vi "Generate_REF_Waveforms.vi"(8 "error in (no error)":errorcluster, 9 "sampling info":cluster{"Fs":dbl, "#s":dbl}={"Fs"=1000.0, "#s"=1000.0} {"Fs" format="%.2p"}, 10 "reset signal":bool, 11 "lockin config":T1 {"TC (s)" format="%#_13g"}) -> (0 "error out":errorcluster, 2 "REF Waveforms":waveform(dbl)[](array[waveform]))   [LabVIEW 2020, in "DSP_lockin.lvclass"]
uses:
  DSP_lockin.lvclass
  Typedefs/Lockin_Config.ctl
  <vilib>/measure/NI_MABase.lvlib
panel:
  out "Numeric":i32
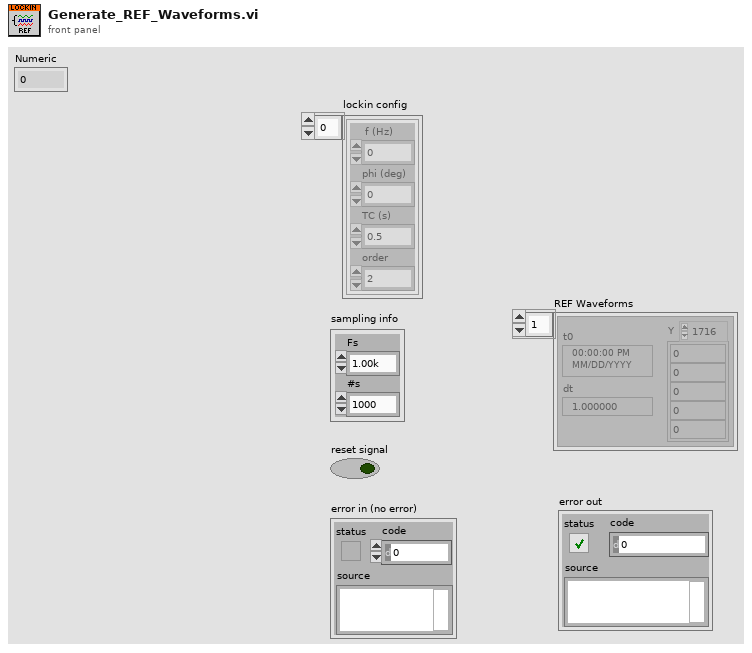
[diagram p1: front panel]
types:
  T1 = typedef "DSP_lockin.lvclass/Lockin_Config.ctl" = cluster{" f (Hz)":dbl, "phi (deg)":dbl, "TC (s)":dbl, "order":i32}[]
  T2 = enum16{"Sine Wave", "Triangle Wave", "Square Wave", "Sawtooth Wave"}
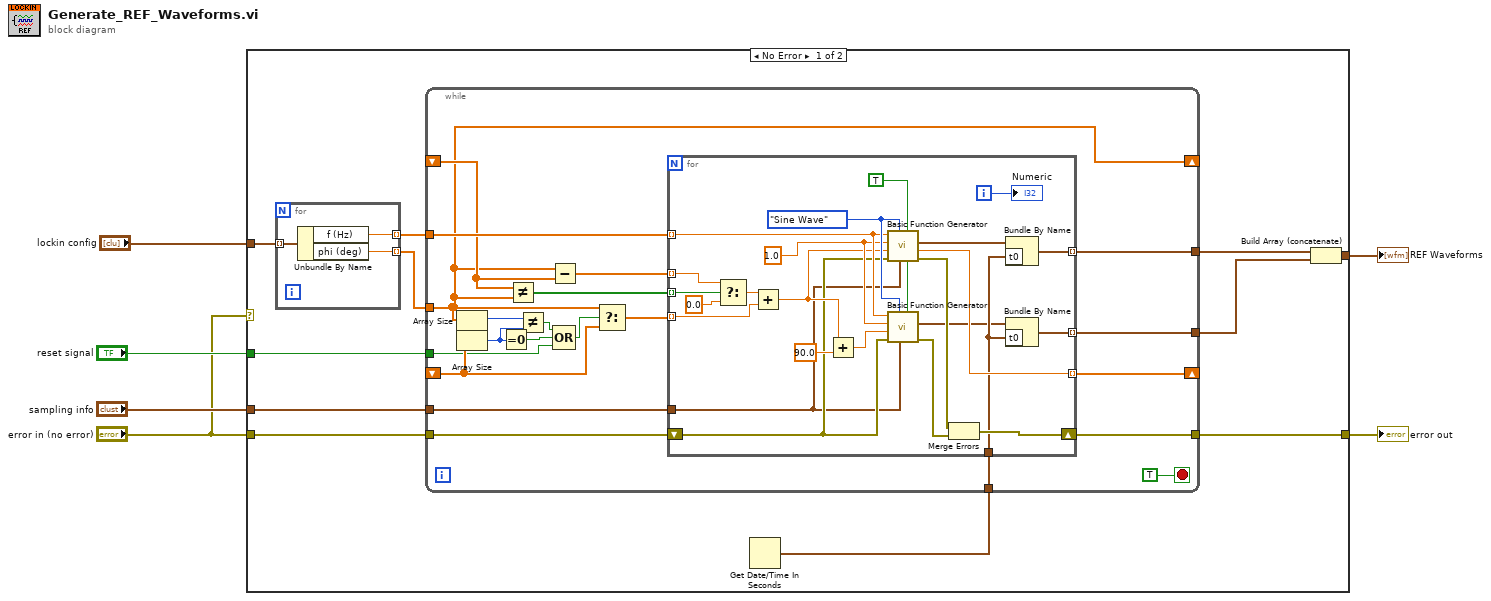
[diagram p0: block diagram]
diagram:
  n1 = case shown="No Error" "error in (no error)" {
    tunnel: [w17 _] -> w6
    tunnel: "reset signal" -> [w14 _]
    tunnel: "sampling info" -> [w13 _]
    tunnel: "error in (no error)" -> [w12 w66]
    tunnel: [w8 w66] -> w3
    tunnel: "lockin config" -> [w7 _]
    frame No Error {
      n2 = for {
        tunnel: w7 -> [w65] mode=indexing
        tunnel: [w64] -> w16 mode=indexing
        tunnel: [w63] -> w15 mode=indexing
        n3 = Unbundle By Name(w65) -> ("f (Hz)"=w64:dbl, "phi (deg)"=w63:dbl)
      }
      n4 = Get Date/Time In Seconds() -> (seconds since 1Jan1904=w11:timestamp)
      n5 = while {
        tunnel: w13 -> [w26]
        tunnel: [w38] -> w10
        tunnel: w15 -> [w22]
        tunnel: w16 -> [w37]
        shift-right: [w22] -> _
        shift-left: _ -> [w35]
        shift-right: [w33] -> _
        shift-left: _ -> [w29]
        tunnel: w11 -> [w32]
        tunnel: w14 -> [w27]
        tunnel: w12 -> [w25]
        tunnel: [w24] -> w8
        tunnel: [w23] -> w9
        stop <- TRUE stop-if-true
        n6 = Array Size(array=w22) -> (size(s)=w20:i32)
        n7 = Array Size(array=w29) -> (size(s)=w19:i32)
        n8 = Equal To 0?(x=w19) -> (x = 0?=w28:bool)
        n9 = Not Equal?(x=w35, y=w22) -> (x != y?=w21:bool[])
        n10 = Not Equal?(x=w20, y=w19) -> (x != y?=w18:bool)
        n11 = Subtract(x=w22, y=w35) -> (x-y=w34:dbl[])
        n12 = Compound Arithmetic op=OR(w18, w28, w27) -> (w31:bool)
        n13 = Select(t=w22, s=w31, f=w29) -> (s? t:f=w30:dbl[])
        n14 = for {
          tunnel: w37 -> [w52] mode=indexing
          tunnel: [w56] -> w38 mode=indexing
          tunnel: w26 -> [w43]
          tunnel: w21 -> [w58] mode=indexing
          tunnel: w34 -> [w60] mode=indexing
          tunnel: [w55] -> w33 mode=indexing
          tunnel: w30 -> [w54] mode=indexing
          tunnel: w32 -> [w41]
          shift-right: [w42] -> w24
          shift-left: w25 -> [w46]
          tunnel: [w39] -> w23 mode=indexing
          i -> [w57]
          w53 = T2."Sine Wave" ("signal type")
          w50 = 1.0 ("amplitude")
          w51 = TRUE ("reset signal")
          n15 = Select(t=w60, s=w58, f=0.0) -> (s? t:f=w61:dbl)
          n16 = Add(x=w61, y=w54) -> (x+y=w49:dbl)
          n17 = Add(x=w49, y=90.0) -> (x+y=w47:dbl)
          n18 = call <vilib>:"Basic Function Generator.vi"("reset signal"=w51, "sampling info"=w43, "signal type"=w53, "error in (no error)"=w46, "phase"=w49, "amplitude"=w50, "frequency"=w52) -> ("error out"=w44:errorcluster, "phase out"=w55:dbl, "signal out"=w62:waveform(dbl))  [unwired: 2 in]
          n19 = call <vilib>:"Basic Function Generator.vi"("reset signal"=w51, "sampling info"=w43, "signal type"=w53, "error in (no error)"=w46, "phase"=w47, "amplitude"=w50, "frequency"=w52) -> ("error out"=w45:errorcluster, "signal out"=w40:waveform(dbl))  [unwired: 2 in, 1 out]
          n20 = Merge Errors(w44, w45) -> (w42:errorcluster)
          n21 = Bundle By Name(cluster=w62, "t0"=w41) -> (w56:waveform(dbl))
          n22 = Bundle By Name(cluster=w40, "t0"=w41) -> (w39:waveform(dbl))
          "Numeric" <- w57
        }
      }
      n23 = Build Array (concatenate)(w10, w9) -> (w17:waveform(dbl)[])
    }
    frame Error {
    }
  }
  "REF Waveforms" <- w6
  "error out" <- w3
